vi "SetConfiguration.vi"(8 "error in (no error)":errorcluster, 11 "Motor Base in":refnum<class "Motor Base.lvclass">) -> (0 "error out":errorcluster, 3 "Motor Base out":refnum<class "Motor Base.lvclass">)   [LabVIEW 2016, in "Motor Base.lvlib" / "Motor Base.lvclass"]
uses:
  Motor Base.lvclass
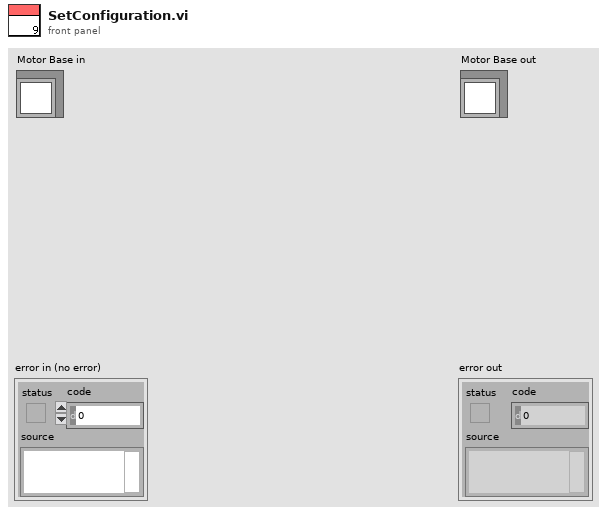
[diagram p1: front panel]
types:
  T1 = cluster{"Modes of operation":i8, "Feed(pulse)":u32, "Max motor speed(r/min)":u32, "Max torque(0.1%)":u16, "Min position limit(pulse)":i32, "Max position limit(pulse)":i32}
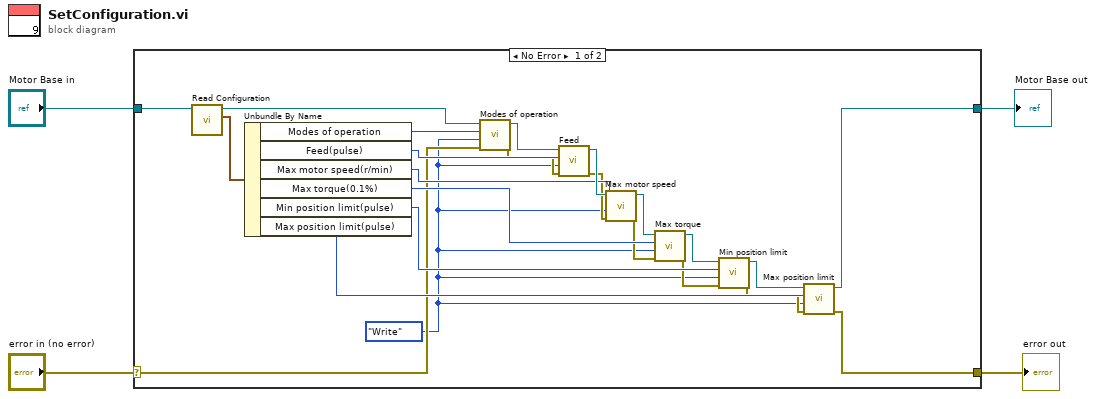
[diagram p0: block diagram]
diagram:
  n1 = case shown="No Error" "error in (no error)" {
    selector: "error in (no error)" -> [w13 w29]
    tunnel: [w7 w29] -> w3
    tunnel: [w6 w28] -> w1
    tunnel: "Motor Base in" -> [w27 w28]
    frame No Error {
      w5 = enum16{"Write", "Read"}."Write" ("W/R")
      n2 = call-dynamic "Read Configuration.vi"("Motor Base in"=w27) -> ("Configuration"=w26:T1, "Motor Base out"=w24:refnum<class "Motor Base.lvclass">)  [unwired: 8 in, 1 out]
      n3 = Unbundle By Name(w26) -> ("Modes of operation"=w25:i8, "Feed(pulse)"=w23:u32, "Max motor speed(r/min)"=w20:u32, "Max torque(0.1%)"=w18:u16, "Min position limit(pulse)"=w16:i32, "Max position limit(pulse)"=w14:i32)
      n4 = call-dynamic "Modes of operation.vi"("error in (no error)"=w13, "W/R"=w5, "Ring"=w25, "Motor Base in"=w24) -> ("error out"=w12:errorcluster, "Motor Base out"=w22:refnum<class "Motor Base.lvclass">)  [unwired: 5 in, 1 out]
      n5 = call-dynamic "Feed.vi"("error in (no error)"=w12, "W/R"=w5, "Feed"=w23, "Motor Base in"=w22) -> ("error out"=w11:errorcluster, "Motor Base out"=w21:refnum<class "Motor Base.lvclass">)  [unwired: 5 in, 1 out]
      n6 = call-dynamic "Max motor speed.vi"("error in"=w11, "W/R"=w5, "Data"=w20, "Motor Base in"=w21) -> ("error out"=w10:errorcluster, "Motor Base out"=w19:refnum<class "Motor Base.lvclass">)  [unwired: 5 in, 1 out]
      n7 = call-dynamic "Max torque.vi"("error in"=w10, "W/R"=w5, "Data"=w18, "Motor Base in"=w19) -> ("error out"=w9:errorcluster, "Motor Base out"=w17:refnum<class "Motor Base.lvclass">)  [unwired: 5 in, 1 out]
      n8 = call-dynamic "Min position limit.vi"("error in (no error)"=w9, "W/R"=w5, "Data"=w16, "Motor Base in"=w17) -> ("error out"=w8:errorcluster, "Motor Base out"=w15:refnum<class "Motor Base.lvclass">)  [unwired: 6 in]
      n9 = call-dynamic "Max position limit.vi"("error in (no error)"=w8, "W/R"=w5, "Data"=w14, "Motor Base in"=w15) -> ("error out"=w7:errorcluster, "Motor Base out"=w6:refnum<class "Motor Base.lvclass">)  [unwired: 6 in]
    }
    frame Error {
    }
  }
  "error out" <- w3
  "Motor Base out" <- w1
